vi "Color_Globals.vi"() -> ()   [LabVIEW 2022 SP3]
panel:
  in  "Text":u32(colorbox)
  in  "Triple Quote":u32(colorbox)=9306312
  in  "Comment":u32(colorbox)=15665920
  in  "Python":u32(colorbox)=11817216
  in  "function":u32(colorbox)=239
  in  "Quote":u32(colorbox)=46086
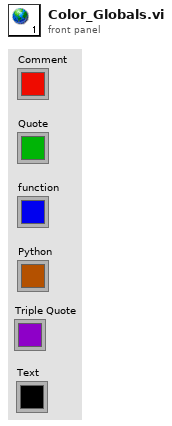
[diagram p1: front panel]
diagram:
